vi "printDaqFunctionBlock.vi"(8 "error in":errorcluster, 9 "Indent":i32, 10 "TreeRef":refnum<vi>, 11 "baseObject in":refnum<class "IBaseObject.lvclass">) -> (0 "error out":errorcluster, 3 "baseObject out":refnum<class "IBaseObject.lvclass">)   [LabVIEW 2022 SP3, in "openDAQ.lvlib" / "daqUtils.lvlib" / "Tree.lvlib"]
uses:
  Tree.lvlib
  IFunctionBlock/IFunctionBlock.lvclass
  IInputPort/IInputPort.lvclass
  ISignal/ISignal.lvclass
  IBaseObject/IBaseObject.lvclass
  IBaseObject/Polymorphic/queryInterface/queryFunctionBlockInterface.vi
  IComponent/IComponent.lvclass
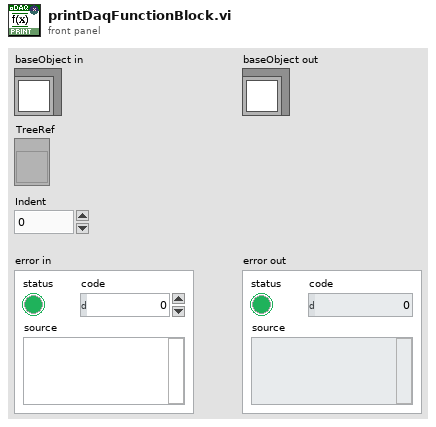
[diagram p1: front panel]
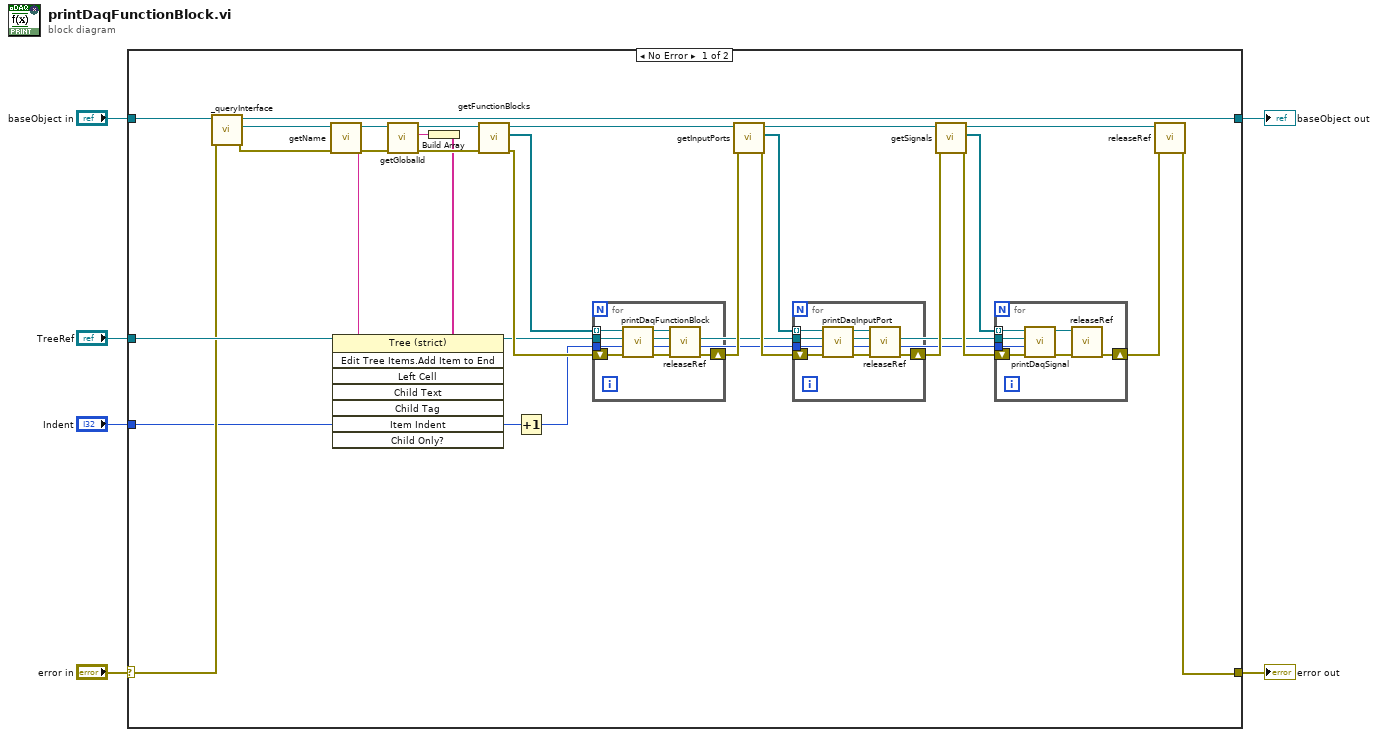
[diagram p0: block diagram]
diagram:
  n1 = case shown="No Error" "error in" {
    selector: "error in" -> [w30 w55]
    tunnel: "baseObject in" -> [w35 w54]
    tunnel: "Indent" -> [w26 _]
    tunnel: "TreeRef" -> [w31 _]
    tunnel: [w29 w55] -> w2
    tunnel: [w33 w54] -> w1
    frame No Error {
      n2 = call-poly "_queryInterface.vi"("error in (no error)"=w30, "IBaseObject in"=w35) -> ("error out"=w32:errorcluster, "IFunctionBlock out"=w34:refnum<class "IFunctionBlock.lvclass">, "IBaseObject out"=w33:refnum<class "IBaseObject.lvclass">)  [unwired: 7 in]
      n3 = call "getName.vi"("error in (no error)"=w32, "IComponent in"=w34) -> ("error out"=w11:errorcluster, "Name out"=w9:string, "IComponent out"=w13:refnum<class "IFunctionBlock.lvclass">)  [unwired: 7 in]
      n4 = call "getGlobalId.vi"("error in (no error)"=w11, "IComponent in"=w13) -> ("error out"=w10:errorcluster, "GlobalId out"=w8:string, "IComponent out"=w12:refnum<class "IFunctionBlock.lvclass">)  [unwired: 7 in]
      n5 = Build Array(w8) -> (w7:string[])
      n6 = invoke class="Tree (strict)" method="Edit Tree Items.Add Item to End"(reference=w31, "Left Cell"=w9, "Child Text"=w7, "Item Indent"=w26) -> (reference out=w16:refnum<vi>)  [unwired: 4 in, 7 out]
      n7 = call "getFunctionBlocks.vi"("error in (no error)"=w10, "IFunctionBlock in"=w12) -> ("error out"=w28:errorcluster, "IFunctionBlocks out"=w27:refnum<class "IFunctionBlock.lvclass">[], "IFunctionBlock out"=w25:refnum<class "IFunctionBlock.lvclass">)  [unwired: 7 in]
      n8 = Increment(x=w26) -> (x+1=w15:i32)
      n9 = for {
        tunnel: w27 -> [w51] mode=indexing
        shift-right: [w52] -> w24
        shift-left: w28 -> [w53]
        tunnel: w16 -> [w49]
        tunnel: w15 -> [w48]
        n10 = call "printDaqFunctionBlock.vi"("Indent"=w48, "TreeRef"=w49, "baseObject in"=w51) -> ("baseObject out"=w50:refnum<class "IFunctionBlock.lvclass">)  [unwired: 7 in, 1 out]
        n11 = call-dynamic "releaseRef.vi"("error in (no error)"=w53, "IBaseObject in"=w50) -> ("error out"=w52:errorcluster)  [unwired: 9 in]
      }
      n12 = call "getInputPorts.vi"("error in (no error)"=w24, "IFunctionBlock in"=w25) -> ("error out"=w23:errorcluster, "IInputPorts out"=w22:refnum<class "IInputPort.lvclass">[], "IFunctionBlock out"=w21:refnum<class "IFunctionBlock.lvclass">)  [unwired: 7 in]
      n13 = for {
        tunnel: w22 -> [w45] mode=indexing
        shift-right: [w46] -> w19
        shift-left: w23 -> [w47]
        tunnel: w16 -> [w43]
        tunnel: w15 -> [w42]
        n14 = call "printDaqInputPort.vi"("Indent"=w42, "TreeRef"=w43, "baseObject in"=w45) -> ("baseObject out"=w44:refnum<class "IInputPort.lvclass">)  [unwired: 7 in, 1 out]
        n15 = call-dynamic "releaseRef.vi"("error in (no error)"=w47, "IBaseObject in"=w44) -> ("error out"=w46:errorcluster)  [unwired: 9 in]
      }
      n16 = call "getSignals.vi"("error in (no error)"=w19, "IFunctionBlock in"=w21) -> ("error out"=w18:errorcluster, "ISignals out"=w17:refnum<class "ISignal.lvclass">[], "IFunctionBlock out"=w20:refnum<class "IFunctionBlock.lvclass">)  [unwired: 7 in]
      n17 = for {
        tunnel: w17 -> [w39] mode=indexing
        shift-right: [w40] -> w14
        shift-left: w18 -> [w41]
        tunnel: w16 -> [w37]
        tunnel: w15 -> [w36]
        n18 = call "printDaqSignal.vi"("Indent"=w36, "TreeRef"=w37, "baseObject in"=w39) -> ("baseObject out"=w38:refnum<class "ISignal.lvclass">)  [unwired: 7 in, 1 out]
        n19 = call-dynamic "releaseRef.vi"("error in (no error)"=w41, "IBaseObject in"=w38) -> ("error out"=w40:errorcluster)  [unwired: 9 in]
      }
      n20 = call-dynamic "releaseRef.vi"("error in (no error)"=w14, "IBaseObject in"=w20) -> ("error out"=w29:errorcluster)  [unwired: 9 in]
    }
    frame Error {
    }
  }
  "error out" <- w2
  "baseObject out" <- w1
